vi "Main.vi"(8 "error in":errorcluster, 11 "DataSave Worker in":refnum<class "DataSave Worker.lvclass">) -> (0 "error out":errorcluster, 3 "DataSave Worker out":refnum<class "DataSave Worker.lvclass">)   [LabVIEW 2018, in "DataSave Worker.lvclass"]
doc: "The Queued Message Handler of a Worker."
uses:
  DataSave Worker.lvclass
  <vilib>/Utility/file.llb/Write Delimited Spreadsheet (string).vi
  Initialization Data.ctl
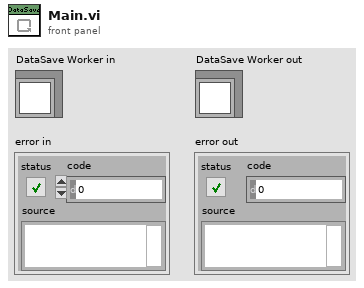
[diagram p1: front panel]
types:
  T1 = typedef "DataSave Worker.lvclass/Initialization Data.ctl" = cluster{"String":string}
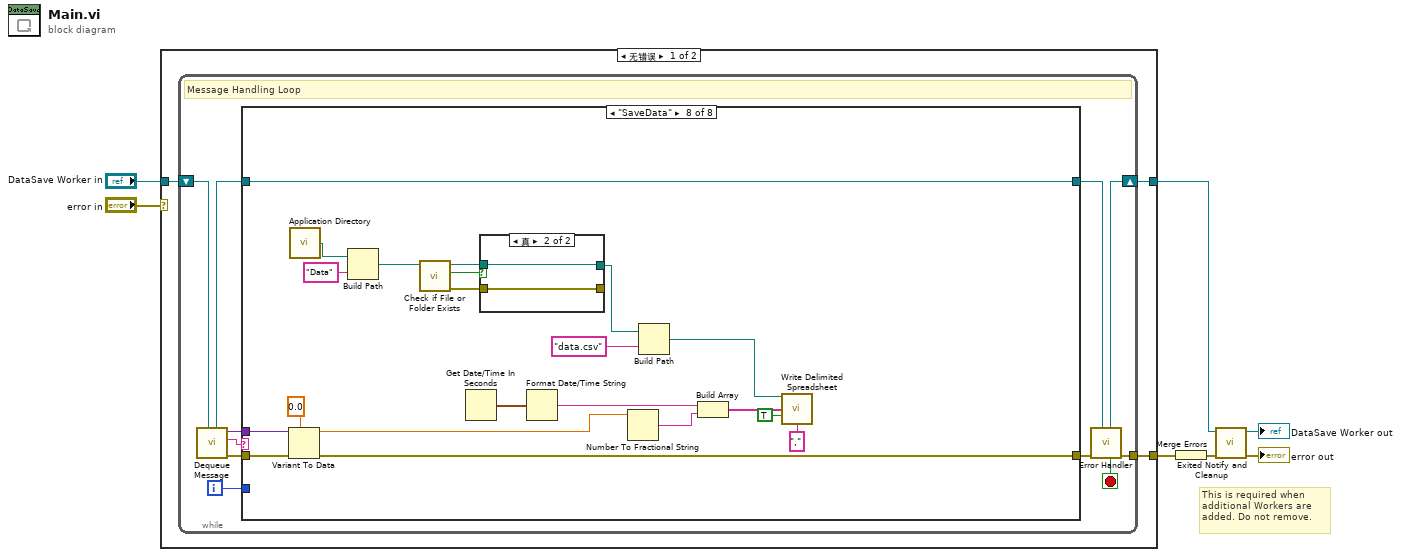
[diagram p0: block diagram]
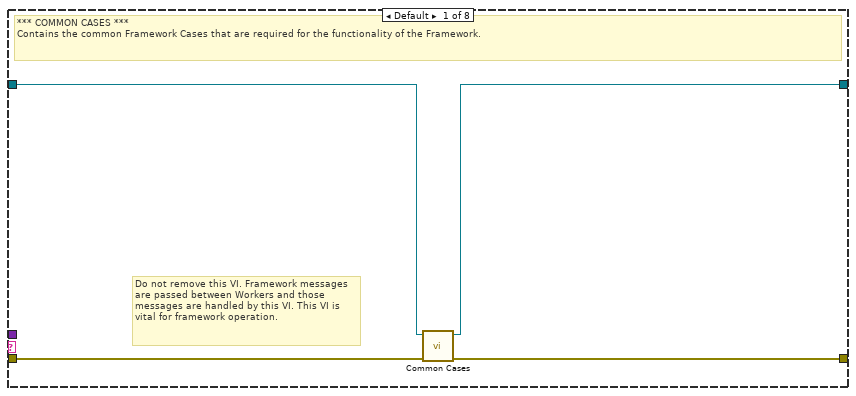
[diagram p2: hidden frame]
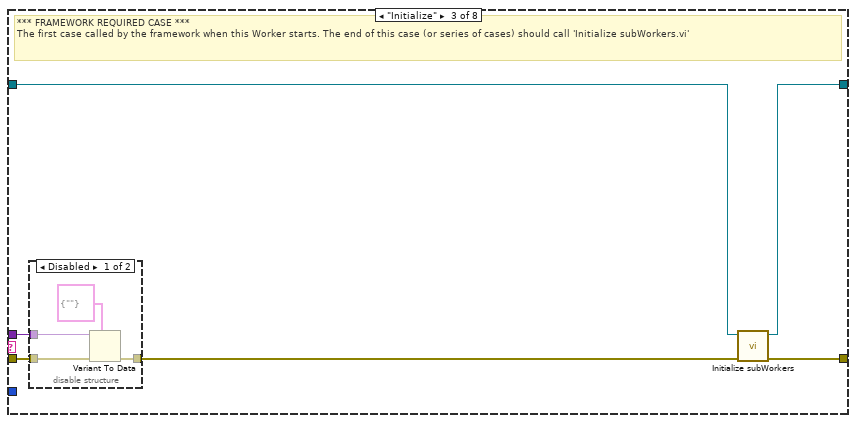
[diagram p4: hidden frame]
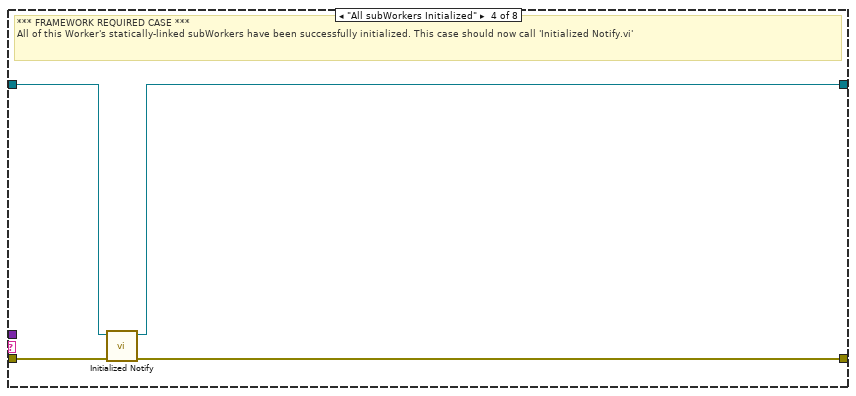
[diagram p6: hidden frame]
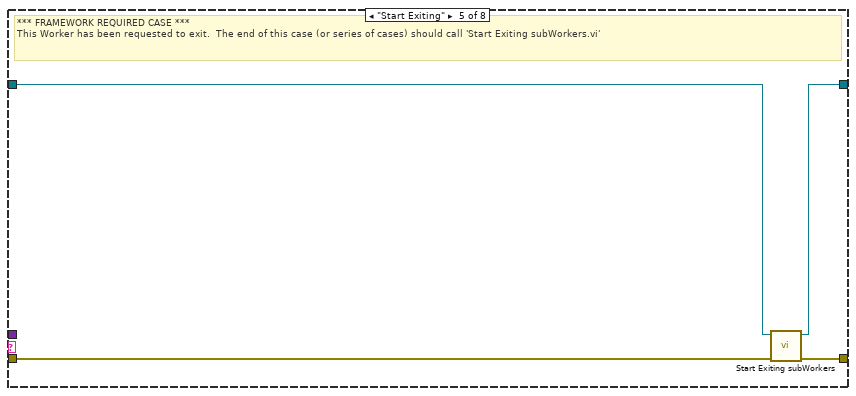
[diagram p7: hidden frame]
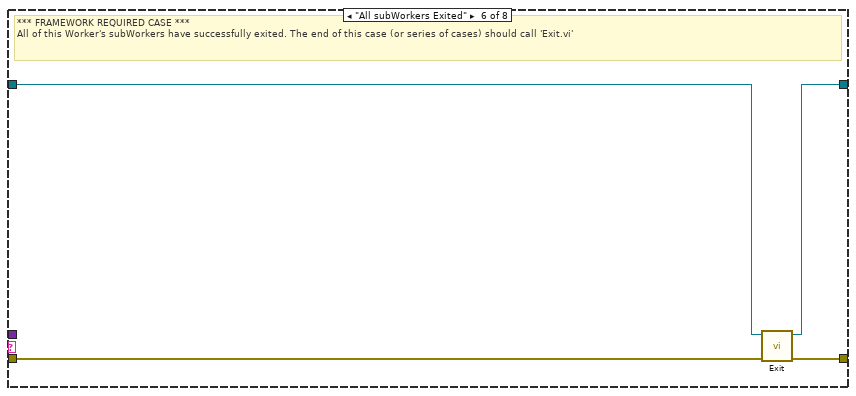
[diagram p8: hidden frame]
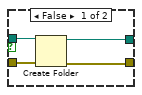
[diagram p10: hidden frame]
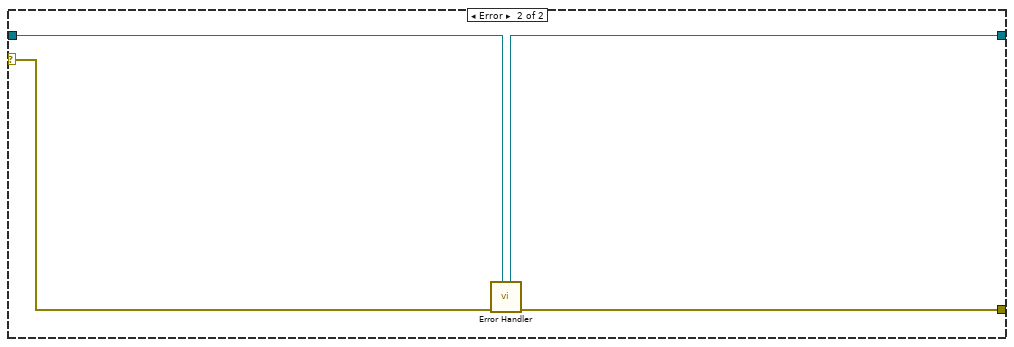
[diagram p11: hidden frame]
diagram:
  # "This is required when additional Workers are added. Do not remove."
  n1 = case shown="无错误" "error in" {
    tunnel: "DataSave Worker in" -> [w8 w81]
    tunnel: [w10 w82] -> w6
    tunnel: [w9 w80] -> w7
    selector: "error in" -> [_ w83]
    frame No Error {
      n2 = while {
        shift-right: [w19] -> w9
        shift-left: w8 -> [w21]
        tunnel: [w20] -> w10
        i -> [w11]
        stop <- w12 stop-if-true
        # "Message Handling Loop"
        n3 = call-dynamic "Dequeue Message.vi"("Worker"=w21) -> ("error out"=w18:errorcluster, "Case out"=w13:string, "Data out"=w14:variant, "Worker out"=w16:refnum<class "DataSave Worker.lvclass">)  [unwired: 6 in, 1 out]
        n4 = case "Worker MHL Case Structure (DO NOT CHANGE LABEL NAME)" shown="\"SaveData\"" w13 {
          tunnel: w18 -> [w25 w26 w31 w42 w43 w50 w51 w68]
          tunnel: [w24 w26 w33 w41 w46 w49 w51 w67] -> w17
          tunnel: w16 -> [w23 w27 w30 w40 w44 w48 w52 w73]
          tunnel: [w22 w27 w32 w39 w45 w47 w52 w73] -> w15
          tunnel: w14 -> [_ _ w28 _ _ _ _ w70]
          tunnel: w11 -> [_ _ _ _ _ _ _ _]
          frame Default {
            # "Do not remove this VI. Framework messages are passed between Workers and those messages are handled by this VI. This VI is vital for framework operation."
            # "*** COMMON CASES ***\nContains the common Framework Cases that are required for the functionality of the Framework."
            n5 = call-dynamic "Common Cases.vi"("error in"=w25, "Worker in"=w23) -> ("error out"=w24:errorcluster, "Worker out"=w22:refnum<class "DataSave Worker.lvclass">)  [unwired: 8 in]
          }
          frame "------ FRAMEWORK REQUIRED CASES ------" {
            # "Start of Framework Required Cases"
          }
          frame "Initialize" {
            # "*** FRAMEWORK REQUIRED CASE ***\nThe first case called by the framework when this Worker starts. The end of this case (or series of cases) should call 'Initialize subWorkers.vi'"
            n6 = disable-structure shown="Disabled" {
              disable-tunnel: w31 -> [w37 w38]
              disable-tunnel: [w36 w38] -> w29
              disable-tunnel: w28 -> [w34 _]
              frame Disabled {
                n7 = Variant To Data(error in=w37, type=T1 {"String"=""} ("Cluster"), Variant=w34) -> (error out=w36:errorcluster)  [unwired: 1 out]
              }
              frame Enabled {
              }
            }
            n8 = call-dynamic "Initialize subWorkers.vi"("error in"=w29, "Worker"=w30) -> ("error out"=w33:errorcluster, "dup Worker out"=w32:refnum<class "DataSave Worker.lvclass">)  [unwired: 8 in]
          }
          frame "All subWorkers Initialized" {
            # "*** FRAMEWORK REQUIRED CASE ***\nAll of this Worker's statically-linked subWorkers have been successfully initialized. This case should now call 'Initialized Notify.vi'"
            n9 = call-dynamic "Initialized Notify.vi"("error in"=w42, "Worker"=w40) -> ("error out"=w41:errorcluster, "dup Worker out"=w39:refnum<class "DataSave Worker.lvclass">)  [unwired: 8 in]
          }
          frame "Start Exiting" {
            # "*** FRAMEWORK REQUIRED CASE ***\nThis Worker has been requested to exit.  The end of this case (or series of cases) should call 'Start Exiting subWorkers.vi'"
            n10 = call-dynamic "Start Exiting subWorkers.vi"("error_in"=w43, "Worker"=w44) -> ("error out"=w46:errorcluster, "dup Worker out"=w45:refnum<class "DataSave Worker.lvclass">)  [unwired: 8 in]
          }
          frame "All subWorkers Exited" {
            # "*** FRAMEWORK REQUIRED CASE ***\nAll of this Worker's subWorkers have successfully exited. The end of this case (or series of cases) should call 'Exit.vi'"
            n11 = call-dynamic "Exit.vi"("error_in"=w50, "Worker"=w48) -> ("error out"=w49:errorcluster, "dup Worker out"=w47:refnum<class "DataSave Worker.lvclass">)  [unwired: 8 in]
          }
          frame "-----------------------------------------------" {
            # "End of Framework Required Cases"
          }
          frame "SaveData" {
            n12 = Variant To Data(error in=w68, type=0.0, Variant=w70) -> (data=w65:dbl, error out=w67:errorcluster)
            n13 = call <vilib>:"Application Directory.vi"() -> ("Application Directory"=w72:path)
            n14 = Build Path(base path=w72, name or relative path="Data" ("名称或相对路径")) -> (appended path=w59:path)
            n15 = call <vilib>:"Check if File or Folder Exists.vi"("path"=w59) -> ("error out"=w56:errorcluster, "file or folder exists?"=w58:bool, "dup path"=w57:path)  [unwired: 8 in]
            n16 = Get Date/Time In Seconds() -> (seconds since 1Jan1904=w66:timestamp)
            n17 = case shown="真" w58 {
              tunnel: w57 -> [w77 w78]
              tunnel: w56 -> [w76 w79]
              tunnel: [w74 w79] -> _
              tunnel: [w75 w78] -> w54
              frame False {
                n18 = Create Folder(path (use dialog)=w77, error in=w76) -> (created path=w75:path, error out=w74:errorcluster)  [unwired: 1 in, 1 out]
              }
              frame True {
              }
            }
            n19 = Format Date/Time String(seconds (now)=w66) -> (date/time string=w64:string)  [unwired: 2 in]
            n20 = Number To Fractional String(number=w65) -> (F-format string=w63:string)  [unwired: 3 in]
            n21 = Build Path(base path=w54, name or relative path="data.csv" ("名称或相对路径")) -> (appended path=w55:path)
            n22 = Build Array(w64, w63) -> (w62:string[])
            n23 = call-poly <vilib>:"Write Delimited Spreadsheet.vi"("file path (dialog if empty)"=w55, "1D data"=w62, "append to file? (new file:F)"=TRUE, "delimiter (\\t)"="," ("delimiter (\\t)")) -> ()  [unwired: 10 in, 2 out]
          }
        }
        n24 = call-dynamic "Error Handler.vi"("Worker"=w15, "error_in"=w17) -> ("error out"=w20:errorcluster, "Stop Loop"=w12:bool, "Worker out"=w19:refnum<class "DataSave Worker.lvclass">)  [unwired: 7 in]
      }
    }
    frame Error {
      n25 = call-dynamic "Error Handler.vi"("Worker"=w81, "error_in"=w83) -> ("error out"=w82:errorcluster, "Worker out"=w80:refnum<class "DataSave Worker.lvclass">)  [unwired: 7 in, 1 out]
    }
  }
  n26 = Merge Errors(w6) -> (w3:errorcluster)
  n27 = call-dynamic "Exited Notify and Cleanup.vi"("error_in"=w3, "Worker"=w7) -> ("error out"=→"error out":errorcluster, "dup Worker out"=→"DataSave Worker out":refnum<class "DataSave Worker.lvclass">)  [unwired: 8 in]
